vi "Turn Off All Outputs.vi"(8 "error in (no error)":errorcluster, 11 "NI-DAQ in":refnum<class "NI-DAQ.lvclass">) -> (0 "error out":errorcluster, 3 "NI-DAQ out":refnum<class "NI-DAQ.lvclass">)   [LabVIEW 2021, in "NI-DAQ.lvclass"]
uses:
  NI-DAQ.lvclass
  NI-DAQ.lvclass/NI-DAQ.ctl
  <vilib>/Utility/file.llb/Read Delimited Spreadsheet (string).vi
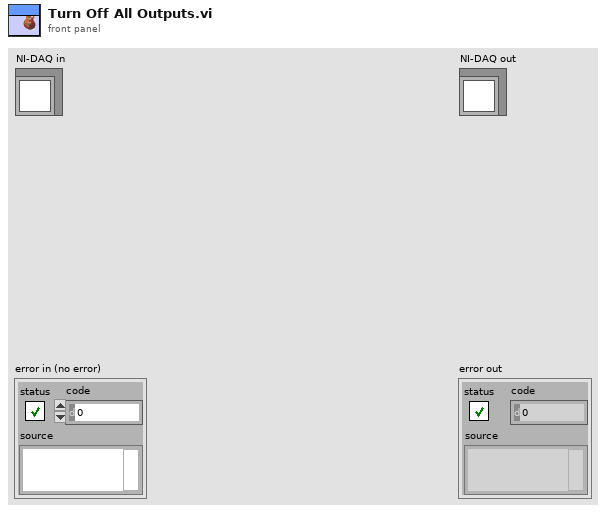
[diagram p1: front panel]
types:
  T1 = typedef "File Paths.ctl" = cluster{"Glue Pattern Folder":path, "Carrier Tray Folder":path, "Pick Up Tool Fixture Folder":path, "Components Folder":path, "Bellows Tool Offset.txt":path, "Pick Up Tool Offset.txt":path, "Dispense Tip Offset.txt":path, "Log Files":path, "Gantry Assembly Map.txt":path, "Syringe and offset map.txt":path, "Controllers Folder":path, "Local dbase config":path}
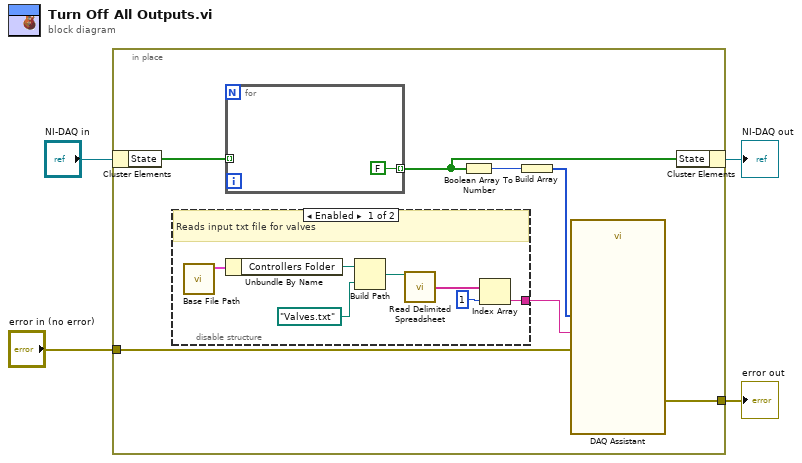
[diagram p0: block diagram]
diagram:
  n1 = in-place {
    in-place-border: [w7] -> w2
    in-place-border: "error in (no error)" -> [w6]
    n2 = in-place-cluster #1("NI-DAQ in") -> ("State"=w11:bool[])
    n3 = disable-structure shown="Enabled" {
      disable-tunnel: [w12 _] -> w5
      frame Enabled {
        # "Reads input txt file for valves"
        n4 = call "Base File Path.vi"() -> ("Paths Out"=w18:T1)  [unwired: 11 in]
        n5 = Unbundle By Name(w18) -> ("Controllers Folder"=w17:path)
        n6 = Build Path(base path=w17, name or relative path=path "Valves.txt") -> (appended path=w15:path)
        n7 = call-poly <vilib>:"Read Delimited Spreadsheet.vi"("file path (dialog if empty)"=w15) -> ("first row"=w14:string[])  [unwired: 9 in, 5 out]
        n8 = Index Array(array=w14, index=1 ("dimension size")) -> (element=w12:string)
      }
      frame Disabled {
      }
    }
    n9 = for {
      tunnel: w11 -> [_] mode=indexing
      tunnel: [FALSE] -> w8 mode=indexing
    }
    n10 = Boolean Array To Number(Boolean array=w8) -> (number=w10:u32)
    n11 = Build Array(w10) -> (w9:u32[])
    n12 = call "DAQ Assistant"("data"=w9, "error in"=w6, "device name"=w5) -> ("error out"=w7:errorcluster)  [unwired: 15 in, 1 out]
    n13 = in-place-cluster #1("State"=w8) -> (→"NI-DAQ out":refnum<class "NI-DAQ.lvclass">)
  }
  "error out" <- w2
